vi "Solution part 2.vi"() -> ()   [LabVIEW 2020]
panel:
  out "error out":errorcluster
  out "result":i64
  in  "data?":bool
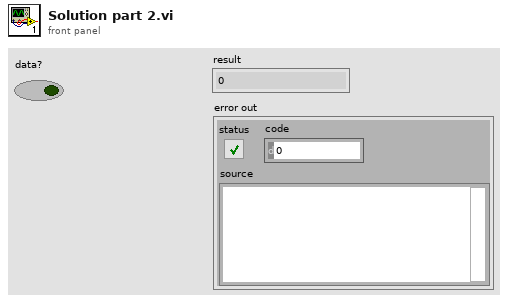
[diagram p1: front panel]
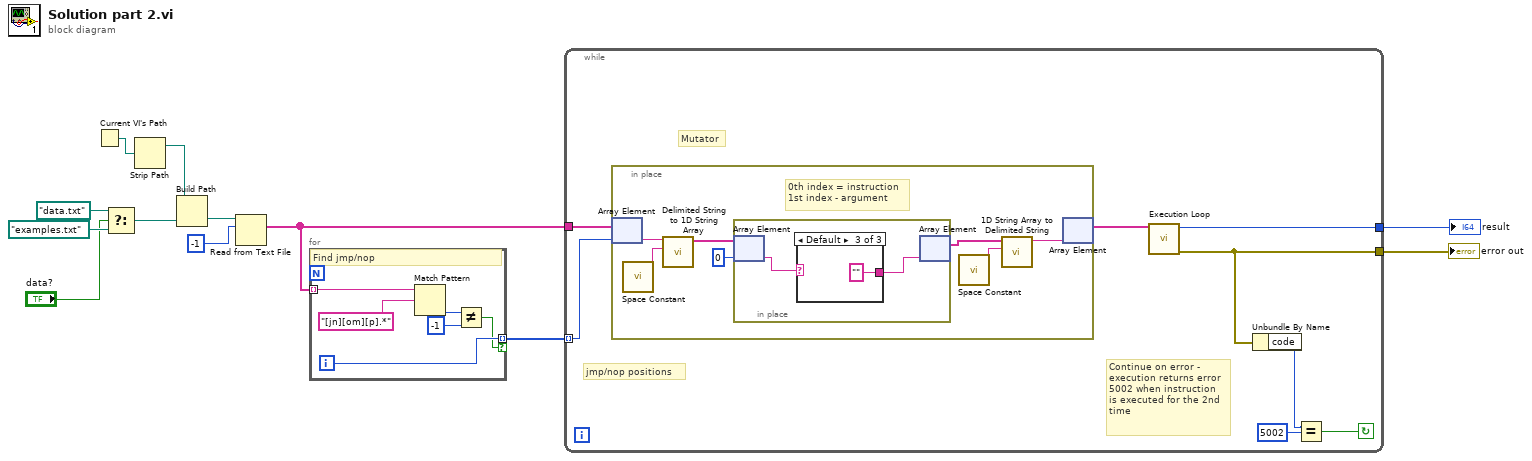
[diagram p0: block diagram]
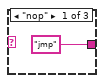
[diagram p2: hidden frame]
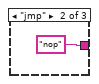
[diagram p3: hidden frame]
diagram:
  n1 = Current VI's Path() -> (path=w8:path)
  n2 = Select(t=path "data.txt", s="data?", f=path "examples.txt") -> (s? t:f=w9:path)
  n3 = Strip Path(path=w8) -> (stripped path=w7:path)  [unwired: 1 out]
  n4 = Build Path(base path=w7, name or relative path=w9) -> (appended path=w6:path)
  n5 = Read from Text File(file (use dialog)=w6, count=-1) -> (text=w2:string[])  [unwired: 2 in, 3 out]
  n6 = for {
    tunnel: w2 -> [w18] mode=indexing
    tunnel: [w14] -> w1 mode=indexing if=w13
    i -> [w14]
    # "Find jmp/nop"
    n7 = Match Pattern(string=w18, regular expression="[jn][om][p].*") -> (offset past match=w16:i32)  [unwired: 1 in, 3 out]
    n8 = Not Equal?(x=w16, y=-1) -> (x != y?=w13:bool)
  }
  n9 = while {
    tunnel: [w25] -> w4
    tunnel: w2 -> [w23]
    tunnel: [w26] -> w3
    tunnel: w1 -> [w22] mode=indexing
    stop <- w21 continue-if-true
    # "jmp/nop positions"
    # "Continue on error - \nexecution returns error\n5002 when instruction\nis executed for the 2nd\ntime"
    # "Mutator"
    n10 = in-place {
      # "0th index = instruction\n1st index - argument"
      n11 = in-place-array #1(w23, w22) -> (w33:string)
      n12 = call <vilib>:"Space Constant.vi"() -> ("String"=w28:string)
      n13 = call <vilib>:"Delimited String to 1D String Array.vi"("delimiter"=w28, "delimited string"=w33) -> ("string array"=w32:string[])  [unwired: 9 in]
      n14 = in-place {
        n15 = in-place-array #2(w32, 0) -> (w35:string)
        n16 = case shown="Default" w35 {
          tunnel: ["jmp" "nop" ""] -> w34
          frame "nop" {
          }
          frame "jmp" {
          }
          frame Default {
          }
        }
        n17 = in-place-array #2(w34) -> (w30:string[])  [unwired: 1 out]
      }
      n18 = call <vilib>:"Space Constant.vi"() -> ("String"=w27:string)
      n19 = call <vilib>:"1D String Array to Delimited String.vi"("delimiter"=w27, "string array"=w30) -> ("delimited string"=w29:string)  [unwired: 9 in]
      n20 = in-place-array #1(w29) -> (w24:string[])  [unwired: 1 out]
    }
    n21 = call "Execution Loop.vi"("Array"=w24) -> ("error out"=w25:errorcluster, "resul"=w26:i64)  [unwired: 9 in]
    n22 = Unbundle By Name(w25) -> ("code"=w20:i32)
    n23 = Equal?(x=w20, y=5002) -> (x = y?=w21:bool)
  }
  "result" <- w3
  "error out" <- w4
